vi "S2C_ExeLoadScript.vi"(8 "Error In":errorcluster) -> (0 "Error Out":errorcluster)   [LabVIEW 2015]
doc: "Loads a script file into the executable table."
uses:
  Globals/S2C_Globals.vi
  <vilib>/Utility/config.llb/Read Key (String).vi
  <vilib>/Utility/config.llb/NI_LVConfig.lvlib
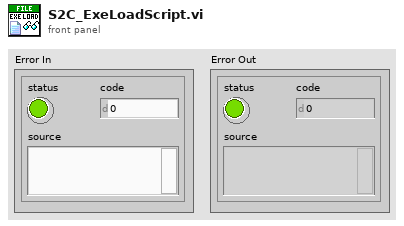
[diagram p1: front panel]
types:
  T1 = typedef "NI_LVConfig.lvlib/Config Data RefNum.ctl" = refnum<k1>
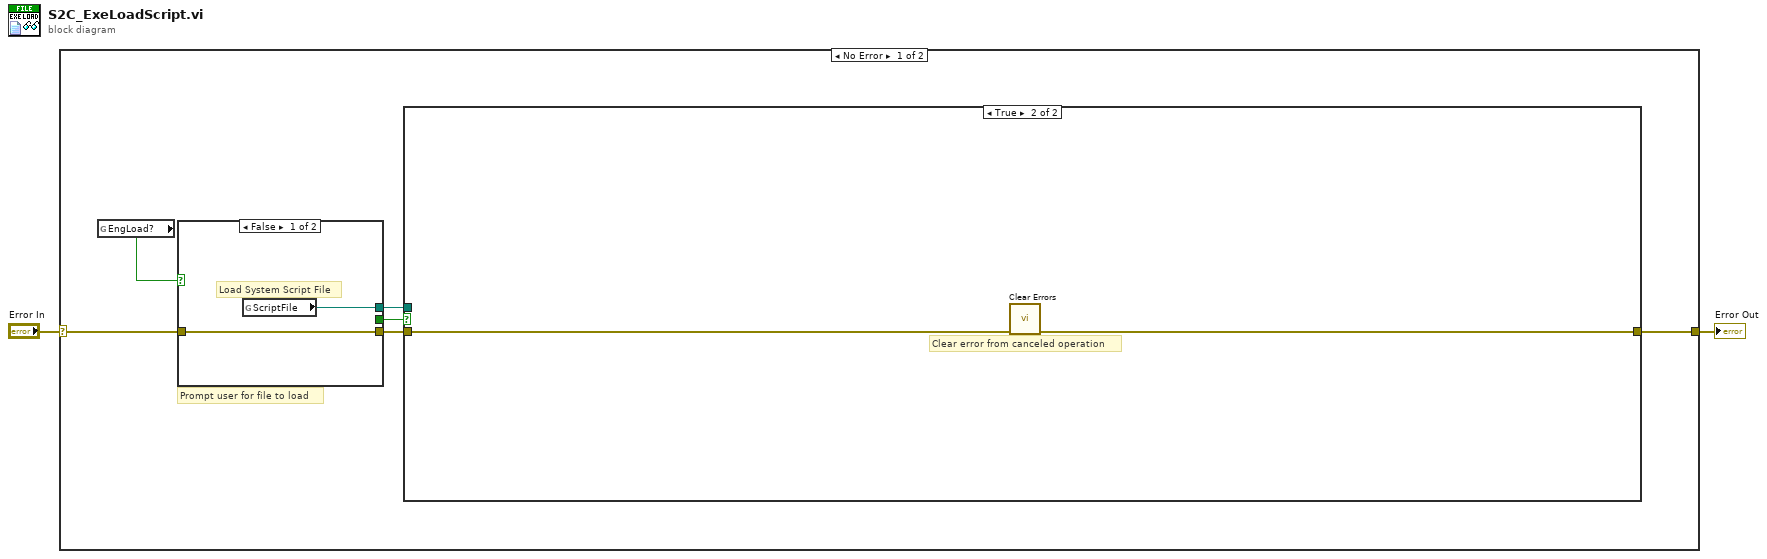
[diagram p0: block diagram]
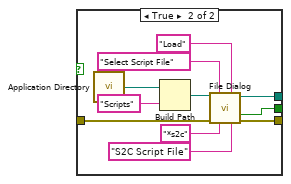
[diagram p2: hidden frame]
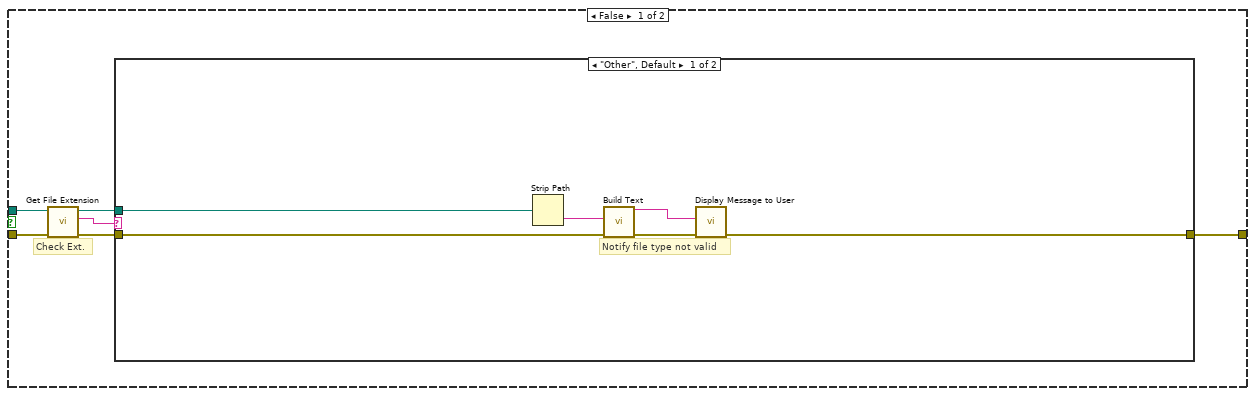
[diagram p3: hidden frame]
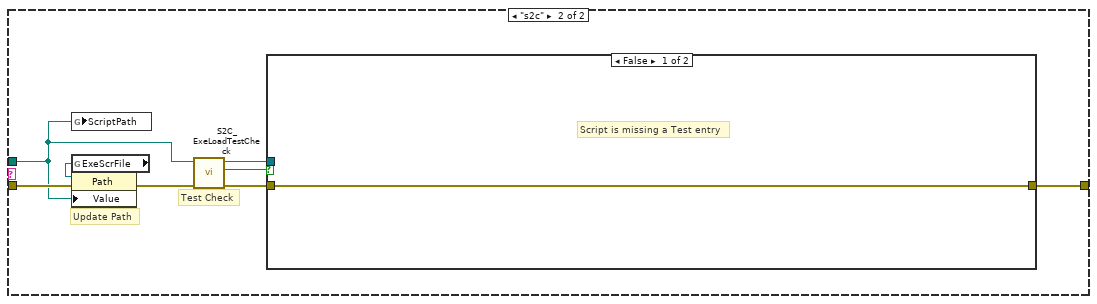
[diagram p4: hidden frame]
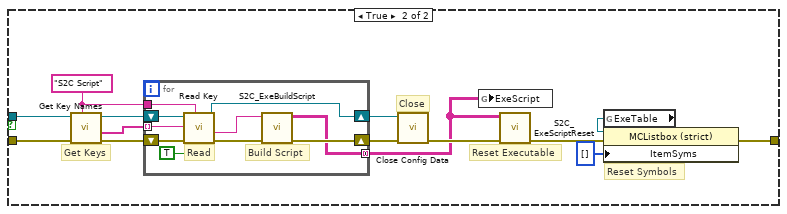
[diagram p5: hidden frame]
diagram:
  n1 = case shown="No Error" "Error In" {
    selector: "Error In" -> [w8 w69]
    tunnel: [w4 w69] -> w1
    frame No Error {
      # "Prompt user for file to load"
      n2 = global read "S2C_Globals.vi" "EngLoad?"() -> (w3:bool)
      n3 = case shown="False" w3 {
        tunnel: w8 -> [w10 w21]
        tunnel: [w10 w13] -> w7
        tunnel: [_ w12] -> w6
        tunnel: [w9 w11] -> w5
        frame False {
          # "Load System Script File"
          n4 = global read "S2C_Globals.vi" "ScriptFile"() -> (w9:path)
        }
        frame True {
          n5 = call <vilib>:"Application Directory.vi"() -> ("Application Directory"=w19:path)
          n6 = Build Path(base path=w19, name or relative path="Scripts") -> (appended path=w17:path)
          n7 = call "File Dialog"("start path"=w17, "prompt"="Select Script File", "button label"="Load", "error in"=w21, "pattern (all files)"="*s2c", "pattern label"="S2C Script File") -> ("selected path"=w11:path, "cancelled"=w12:bool, "error out"=w13:errorcluster)  [unwired: 6 in, 1 out]
        }
      }
      n8 = case shown="True" w6 {
        tunnel: w7 -> [w26 w68]
        tunnel: w5 -> [w24 _]
        tunnel: [w27 w67] -> w4
        frame False {
          # "Check Ext."
          n9 = call <vilib>:"Get File Extension.vi"("error in (no error)"=w26, "file"=w24) -> ("error out"=w25:errorcluster, "lowercase file extension"=w22:string, "dup file"=w23:path)  [unwired: 5 in, 2 out]
          n10 = case shown="\"Other\", Default" w22 {
            tunnel: w25 -> [w30 w40]
            tunnel: [w29 w41] -> w27
            tunnel: w23 -> [w28 w34]
            frame "Other", Default {
              # "Notify file type not valid"
              n11 = Strip Path(path=w28) -> (name=w33:string)  [unwired: 1 out]
              n12 = call "Build Text"("File"=w33, "error in (no error)"=w30) -> ("Result"=w31:string, "error out"=w32:errorcluster)  [unwired: 12 in]
              n13 = call "Display Message to User"("error in (no error)"=w32, "Message"=w31) -> ("error out"=w29:errorcluster)  [unwired: 8 in, 1 out]
            }
            frame "s2c" {
              # "Test Check"
              # "Update Path"
              n14 = global write "S2C_Globals.vi" "ScriptPath"(w34) -> ()
              n15 = global read "S2C_Globals.vi" "ExeScrFile"() -> (w39:refnum<vi>)
              n16 = property class="Path"(reference=w39, error in=w40, "Value"=w34) -> (error out=w35:errorcluster)  [unwired: 1 out]
              n17 = call "S2C_ExeLoadTestCheck.vi"("Error In"=w35, "FilePath"=w34) -> ("Error Out"=w38:errorcluster, "Valid?"=w36:bool, "FileRef Out"=w37:T1)  [unwired: 7 in]
              n18 = case shown="False" w36 {
                tunnel: [w42 w45] -> w41
                tunnel: w38 -> [w42 w44]
                tunnel: w37 -> [_ w43]
                frame False {
                  # "Script is missing a Test entry"
                }
                frame True {
                  w53 = "S2C Script"
                  # "Reset Symbols"
                  # "Reset Executable"
                  # "Get Keys"
                  # "Close"
                  n19 = call <vilib>:"Get Key Names.vi"("section"=w53, "error in (no error)"=w44, "refnum"=w43) -> ("error out"=w54:errorcluster, "key names"=w51:string[], "refnum out"=w52:T1)  [unwired: 5 in, 1 out]
                  n20 = for {
                    shift-right: [w61] -> w56
                    shift-left: w54 -> [w66]
                    tunnel: w53 -> [w65]
                    shift-right: [w58] -> w55
                    shift-left: w52 -> [w64]
                    tunnel: w51 -> [w63] mode=indexing
                    tunnel: [w60] -> w49 mode=concatenating
                    # "Build Script"
                    # "Read"
                    n21 = call-poly <vilib>:"Read Key.vi"("read raw string? (F)"=TRUE, "section"=w65, "error in (no error)"=w66, "key"=w63, "refnum"=w64) -> ("error out"=w62:errorcluster, "value"=w59:string, "refnum out"=w58:T1)  [unwired: 3 in, 1 out]
                    n22 = call "S2C_ExeBuildScript.vi"("Error In"=w62, "Entry"=w59) -> ("Error Out"=w61:errorcluster, "Data"=w60:string[][])  [unwired: 8 in]
                  }
                  n23 = call <vilib>:"Close Config Data.vi"("error in (no error)"=w56, "refnum"=w55) -> ("error out"=w50:errorcluster)  [unwired: 8 in, 1 out]
                  n24 = global write "S2C_Globals.vi" "ExeScript"(w49) -> ()
                  n25 = call "S2C_ExeScriptReset.vi"("Error In"=w50, "Script Data"=w49) -> ("Error Out"=w47:errorcluster)  [unwired: 9 in]
                  n26 = global read "S2C_Globals.vi" "ExeTable"() -> (w48:refnum<vi>)
                  n27 = property on="Property Node" class="MCListbox (strict)"(reference=w48, error in=w47, "ItemSyms"=i32[] [] ("Item Symbols")) -> (error out=w45:errorcluster)  [unwired: 1 out]
                }
              }
            }
          }
        }
        frame True {
          # "Clear error from canceled operation"
          n28 = call <vilib>:"Clear Errors.vi"("error in (no error)"=w68) -> ("error out"=w67:errorcluster)  [unwired: 5 in, 1 out]
        }
      }
    }
    frame Error {
    }
  }
  "Error Out" <- w1
